vi "configuration UI.vi"() -> ()   [LabVIEW 2015, in "tag select module editor node.lvclass"]
uses:
  tag select module editor node.lvclass
  <vilib>/NI/DCAF UI Toolkit/Controls/Remove.ctl
  <vilib>/NI/DCAF UI Toolkit/Controls/Add.ctl
  <vilib>/NI/Configuration Framework/Node/NodeRef.ctl
  <vilib>/NI/Configuration Framework/Node/NISE_CEF_Node.lvclass
  <vilib>/NI/AMC/Message Queue.ctl
  <vilib>/NI/AMC/Message.ctl
  <vilib>/NI/Tools/Keyed Array/KeyedArray.ctl
  <vilib>/NI/Configuration Framework/Node/UserEventRef.ctl
  <vilib>/NI/Configuration Framework/Controls/EventCluster.ctl
  <vilib>/NI/Configuration Framework/Node/StopEvent.ctl
  <vilib>/NI/Configuration Framework/Node/RefreshUIEvent.ctl
  <vilib>/NI/Configuration Framework/Node/CacheState.ctl
  <vilib>/NI/Configuration Framework/Node/NodeChangeEvent.ctl
  <vilib>/NI/Tag Bus/tag/Data Type.ctl
  <vilib>/NI/DCAF/Tag Editor Core/Table API/Available Tag Menu/channel action event.ctl
  <vilib>/NI/DCAF/Tag Editor Core/Table API/Available Tag Menu/dialog output action.ctl
  <vilib>/NI/Tag Bus Module Framework/channel/TBM channel.lvclass
  <vilib>/NI/Tag Bus/tag/tag descriptor.lvclass
  <vilib>/NI/DCAF/Tag Editor Core/Table API/Table Manager/Call Back Ref Type Def.ctl
  <vilib>/NI/DCAF/Tag Editor Core/Configuration Editor/Classes/Engine Parent/Engine Parent Editor Node.lvclass
  <vilib>/NI/DCAF/Tag Editor Core/Configuration Editor/Classes/Module editor node/module editor node.lvclass
  <vilib>/NI/DCAF UI Toolkit/Controls/Import.ctl
  <vilib>/NI/DCAF UI Toolkit/Controls/Export.ctl
  <vilib>/NI/DCAF/Tag Editor Core/Table API/Table Manager/object ref.ctl
  <vilib>/NI/DCAF/Tag Editor Core/Table API/Table Manager/references.ctl
  <vilib>/NI/DCAF/Tag Editor Core/Table API/Listbox/Multi Column Listbox.lvclass
  <vilib>/NI/DCAF/Tag Editor Core/Table API/Listbox/Multi Column Listbox.lvclass/Multi Column Listbox.ctl
  <vilib>/NI/DCAF/Tag Editor Core/Table API/Table Manager/Table Manager.lvclass/Table Manager.ctl
  <vilib>/NI/DCAF/Tag Editor Core/Table API/Listbox/Write Listbox.vi
  <vilib>/NI/DCAF/Tag Editor Core/Table API/Table Manager/Write Top VI.vi
  <vilib>/NI/DCAF/Tag Editor Core/Table API/Table Manager.lvlib
  <vilib>/NI/DCAF/Tag Editor Core/Table API/Table Manager/Table Manager.lvclass
  <vilib>/NI/Tools/Keyed Array/Tools_KeyedArray.lvlib
  <vilib>/NI/AMC/AMC.lvlib
  <vilib>/NI/Configuration Framework/NISE_CEF_TreeControl.lvlib
  <vilib>/NI/DCAF UI Toolkit/Controls/DCAF UI Elements.lvlib
panel:
  in  "dt":T1
  in  "Tab Control":enum32{"Static Configuration", "Import Export"}(tab)
  in  "tag select":i32(listbox)=1
  in  "Add tag select":T2
  in  "remove tag select":T3
  in  "Export":T4
  in  "Import":T5
  in  "user event out":refnum<user-event>
  in  "node change":T6
  in  "cache state":T7
  in  "refresh UI":T8
  in  "stop event":T9
  in  "user event":T10
  in  "main queue":T11
  in  "node ref":T12
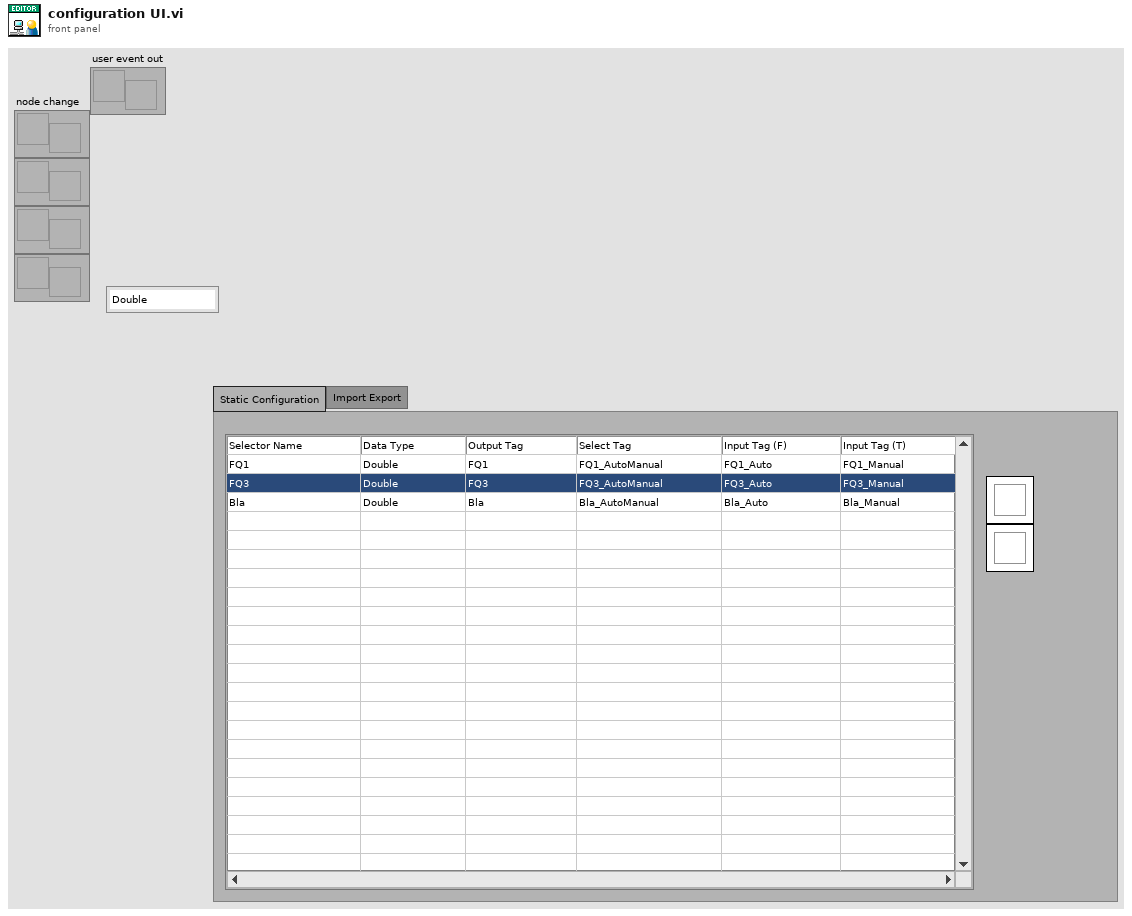
[diagram p1: front panel]
types:
  T1 = typedef "tag bus.lvlib/tag descriptor.lvclass/Data Type.ctl" = enum16{"Double", "Single", "I64", "I32", "I16", "I8", "U64", "U32", "U16", "U8", "Boolean", "String", "Array of Double", "Array of Single", "Array of I64", "Array of I32", "Array of I16", "Array of I8", "Array of U64", "Array of U32", "Array of U16", "Array of U8", "Array of Boolean", "Array of String"}
  T2 = typedef "DCAF UI Elements.lvlib/Add.ctl" = bool
  T3 = typedef "DCAF UI Elements.lvlib/Remove.ctl" = bool
  T4 = typedef "DCAF UI Elements.lvlib/Export.ctl" = bool
  T5 = typedef "DCAF UI Elements.lvlib/Import.ctl" = bool
  T6 = typedef "NISE_CEF_Node.lvclass/NodeChangeEvent.ctl" = refnum<user-event>
  T7 = typedef "NISE_CEF_Node.lvclass/CacheState.ctl" = refnum<user-event>
  T8 = typedef "NISE_CEF_Node.lvclass/RefreshUIEvent.ctl" = refnum<user-event>
  T9 = typedef "NISE_CEF_Node.lvclass/StopEvent.ctl" = refnum<user-event>
  T10 = typedef "NISE_CEF_Node.lvclass/UserEventRef.ctl" = refnum<user-event>
  T11 = typedef "AMC.lvlib/Message Queue.ctl" = refnum<queue>
  T12 = typedef "NISE_CEF_Node.lvclass/NodeRef.ctl" = refnum<data-value>
  T13 = typedef "Table Manager.lvlib/Table Manager.lvclass/references.ctl" = cluster{"stop event":T9, "refresh UI":T8, "cache state":T7, "node change":T6, "user event out":refnum<user-event>, "main queue":T11, "user event":T10}
  T14 = typedef "Table Manager.lvlib/Table Manager.lvclass/object ref.ctl" = cluster{"engine":refnum<data-value>, "Node Ref":refnum<data-value>}
  T15 = typedef "Table Manager.lvlib/Column.lvclass/Column Descriptor.ctl" = cluster{"name":string, "caption":string, "Column Type":T16, "Params":string, "AutoSizeMode":i32, "FillWeight":sgl, "MinWidth":u32, "tooltip":string, "Enum Reference":refnum<vi>, "Channel suffix":string, "Read Only":bool, "Call Back VI":T17, "DT Dependency":i32, "name dependency":i32, "data type":T1, "Custom Column":refnum<class "Column.lvclass">}
  T16 = typedef "Table Manager.lvlib/Column.lvclass/Column Type.ctl" = enum16{"String", "Mapping", "Enum", "Custom"}
  T17 = typedef "Table Manager.lvlib/Table Manager.lvclass/Call Back Ref Type Def.ctl" = refnum<vi>
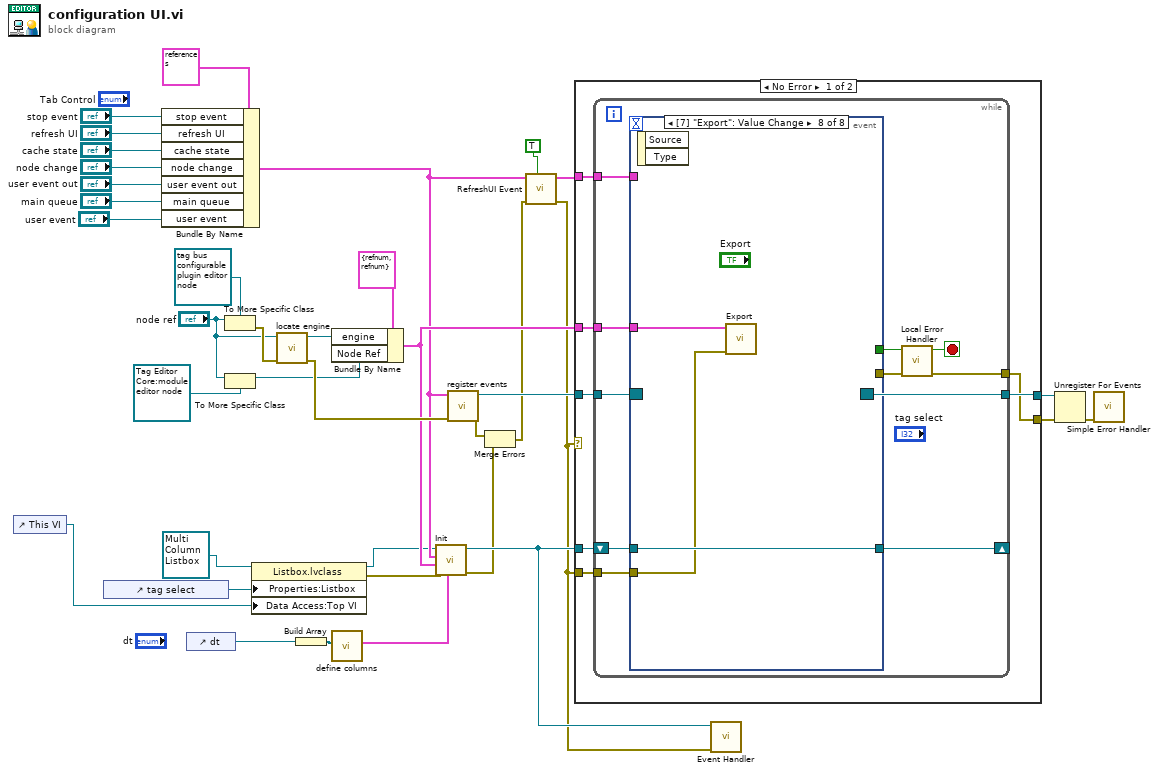
[diagram p0: block diagram]
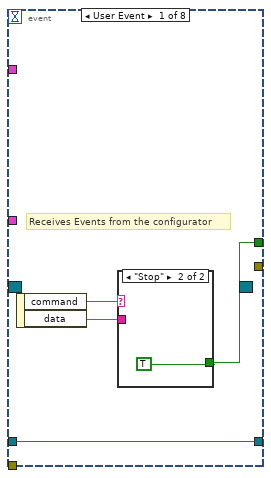
[diagram p2: hidden frame]
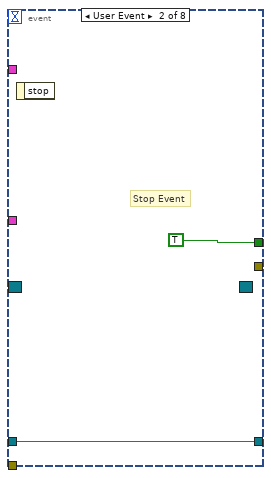
[diagram p4: hidden frame]
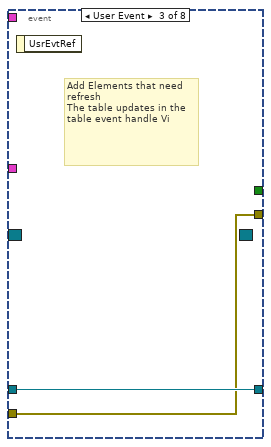
[diagram p5: hidden frame]
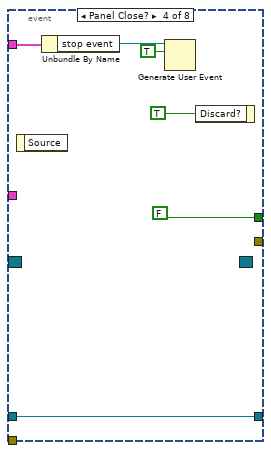
[diagram p6: hidden frame]
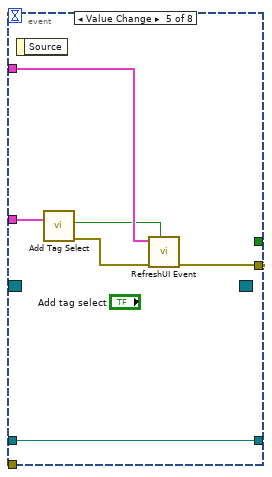
[diagram p7: hidden frame]
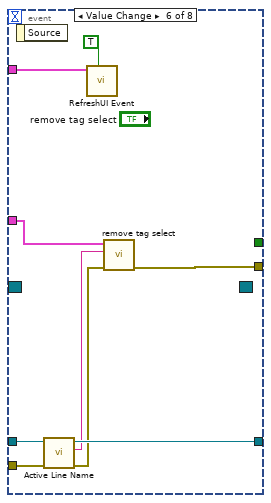
[diagram p8: hidden frame]
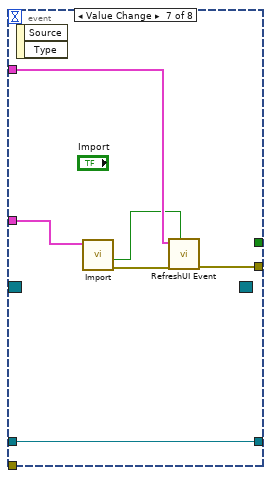
[diagram p9: hidden frame]
diagram:
  n1 = control-ref of="This VI"() -> (w13:refnum<vi>)
  n2 = control-ref of="tag select"() -> (w14:refnum<vi>)
  n3 = Bundle By Name(cluster=T13 {"stop event"=refnum, "refresh UI"=refnum, "cache state"=refnum, "node change"=refnum, "user event out"=refnum, "main queue"=refnum, "user event"=refnum} ("References"), "stop event"="stop event", "refresh UI"="refresh UI", "cache state"="cache state", "node change"="node change", "user event out"="user event out", "main queue"="main queue", "user event"="user event") -> (w9:T13)
  n4 = control-ref of="dt"() -> (w12:refnum<vi>)
  n5 = To More Specific Class(target class=refnum<data-value> refnum ("data value reference"), reference="node ref") -> (error out=w22:errorcluster)  [unwired: 1 in, 1 out]
  n6 = To More Specific Class(target class=refnum<data-value> refnum ("data value reference"), reference="node ref") -> (specific class reference=w2:refnum<data-value>)  [unwired: 1 in, 1 out]
  n7 = property class="Listbox.lvclass"(reference=refnum<class "Multi Column Listbox.lvclass"> refnum ("Table Manager.lvlib:Multi Column Listbox.lvclass"), "Properties:Listbox"=w14, "Data Access:Top VI"=w13) -> (reference out=w1:refnum<class "Multi Column Listbox.lvclass">, error out=w18:errorcluster)  [unwired: 1 in]
  n8 = call <vilib>:"locate engine.vi"("error in"=w22, "component"="node ref") -> ("error out"=w19:errorcluster, "engine"=w21:refnum<data-value>)  [unwired: 8 in]
  n9 = Build Array(w12) -> (w11:refnum<vi>[])
  n10 = Bundle By Name(cluster=T14 {"engine"=refnum, "Node Ref"=refnum} ("references"), "engine"=w21, "Node Ref"=w2) -> (w10:T14)
  n11 = call "define columns.vi"("Enum Array"=w11) -> ("Column Definition"=w17:T15[])  [unwired: 10 in]
  n12 = call-dynamic "Init.vi"("Column Descriptors"=w17, "error in (no error)"=w18, "Node object refs"=w10, "Event References"=w9, "Multi Column Listbox in"=w1) -> ("error out"=w8:errorcluster, "Multi Column Listbox out"=w32:refnum<class "Multi Column Listbox.lvclass">)  [unwired: 4 in, 1 out]
  n13 = call "register events.vi"("error in (no error)"=w19, "References"=w9) -> ("error out"=w7:errorcluster, "Event Registration Refnum"=w34:refnum<event-registration>)  [unwired: 8 in]
  n14 = Merge Errors(w7, w8) -> (w6:errorcluster)
  n15 = call "RefreshUI Event.vi"("Refresh?"=TRUE, "error in"=w6, "References in"=w9) -> ("error out"=w5:errorcluster, "References out"=w33:T13)  [unwired: 7 in]
  n16 = case shown="No Error" w5 {
    selector: w5 -> [_ w96]
    tunnel: w34 -> [w44 w95]
    tunnel: [w43 w95] -> w37
    tunnel: [w42 w96] -> w36
    tunnel: w33 -> [w41 _]
    tunnel: w10 -> [w40 _]
    tunnel: w32 -> [w39 _]
    tunnel: w5 -> [w38 _]
    frame No Error {
      n17 = while {
        tunnel: w44 -> [w55]
        tunnel: [w54] -> w43
        tunnel: [w51] -> w42
        tunnel: w41 -> [w49]
        tunnel: w40 -> [w48]
        shift-right: [w46] -> _
        shift-left: w39 -> [w47]
        tunnel: w38 -> [w45]
        stop <- w53 stop-if-true
        n18 = event shown="[7] \"Export\": Value Change" {
          selector: w55 -> [_ _ _ _ _ _ _ _]
          dyn-events: [_ _ _ _ _ _ _ _] -> w54
          timeout: _ -> [_ _ _ _ _ _ _ _]
          tunnel: [w59 TRUE _ FALSE _ _ _ _] -> w52
          tunnel: [_ _ w63 _ w72 w85 w90 _] -> w50
          tunnel: w49 -> [_ _ _ w66 w75 w83 w89 _]
          tunnel: w48 -> [_ _ _ _ w71 w82 w88 w93]
          tunnel: w47 -> [w56 w61 w64 w65 w76 w81 w91 w94]
          tunnel: [w56 w61 w64 w65 w76 w79 w91 w94] -> w46
          tunnel: w45 -> [_ _ w63 _ _ w80 _ w92]
          event User Event {
            # "Receives Events from the configurator"
            n19 = event-data() -> ("command"=w58:string, "data"=w57:string)  [unwired: 1 in]
            n20 = case shown="\"Stop\"" w58 {
              tunnel: [_ TRUE] -> w59
              tunnel: w57 -> [_ _]
              frame Default {
              }
              frame "Stop" {
              }
            }
          }
          event User Event {
            # "Stop Event"
            n21 = event-data() -> ()  [unwired: 1 in, 1 out]
          }
          event User Event {
            # "Add Elements that need refresh \nThe table updates in the table event handle Vi"
            n22 = event-data() -> ()  [unwired: 1 in, 1 out]
          }
          event Panel Close? {
            n23 = event-data() -> ()  [unwired: 1 in, 1 out]
            n24 = Unbundle By Name(w66) -> ("stop event"=w67:T9)
            n25 = Generate User Event(user event=w67, event data cluster=TRUE ("event data")) -> ()  [unwired: 2 in, 2 out]
            n26 = event-data("Discard?"=TRUE) -> ()  [unwired: 1 in, 1 out]
          }
          event Value Change {
            n27 = event-data() -> ()  [unwired: 1 in, 1 out]
            n28 = call "Add Tag Select.vi"("references"=w71) -> ("error out"=w73:errorcluster, "newtag?"=w74:bool)  [unwired: 9 in]
            n29 = call "RefreshUI Event.vi"("Refresh?"=w74, "error in"=w73, "References in"=w75) -> ("error out"=w72:errorcluster)  [unwired: 7 in, 1 out]
          }
          event Value Change {
            n30 = event-data() -> ()  [unwired: 1 in, 1 out]
            n31 = call-dynamic "Active Line Name.vi"("error in"=w80, "Multi Column Listbox in"=w81) -> ("error out"=w77:errorcluster, "Active Line Name"=w78:string, "Multi Column Listbox out"=w79:refnum<class "Multi Column Listbox.lvclass">)  [unwired: 7 in]
            n32 = call "RefreshUI Event.vi"("Refresh?"=TRUE, "References in"=w83) -> ()  [unwired: 8 in, 2 out]
            n33 = call "remove tag select.vi"("error in"=w77, "tag select"=w78, "object ref in"=w82) -> ("error out"=w85:errorcluster)  [unwired: 8 in]
          }
          event Value Change {
            n34 = event-data() -> ()  [unwired: 1 in, 2 out]
            n35 = call "Import.vi"("Objects in"=w88) -> ("error out"=w86:errorcluster, "Update"=w87:bool)  [unwired: 8 in, 1 out]
            n36 = call "RefreshUI Event.vi"("Refresh?"=w87, "error in"=w86, "References in"=w89) -> ("error out"=w90:errorcluster)  [unwired: 7 in, 1 out]
          }
          event Value Change {
            n37 = event-data() -> ()  [unwired: 1 in, 2 out]
            n38 = call "Export.vi"("error in"=w92, "Objects in"=w93) -> ()  [unwired: 9 in, 1 out]
          }
        }
        n39 = call "Local Error Handler.vi"("error in"=w50, "stop in"=w52) -> ("error out"=w51:errorcluster, "stop out"=w53:bool)  [unwired: 8 in]
      }
    }
    frame Error {
    }
  }
  n40 = call-dynamic "Event Handler.vi"("error in"=w5, "Listbox in"=w32) -> ()  [unwired: 8 in, 2 out]
  n41 = Unregister For Events(event registration refnum=w37, error in=w36) -> (error out=w35:errorcluster)
  n42 = call <vilib>:"Simple Error Handler.vi"("error in (no error)"=w35) -> ()  [unwired: 4 in, 5 out]
